vi "FGV.vi"(8 "error out 2":errorcluster, 10 "Write Data":T1, 11 "Enum":T5) -> (0 "error out":errorcluster, 3 "Read Data":T1)   [LabVIEW 2015, in "Copy of Untitled Library 1.lvlib"]
uses:
  Copy of Untitled Library 1.lvlib
  Controls/Enum Constant.ctl
  Controls/FGV Data.ctl
  Controls/FGV Cluster Data.ctl
  <userlib>/origin_lib_main/userlogin_lib/Control/Queue and Caller MSG.ctl
  <vilib>/addons/database/Connection.llb/Conn ObjectReference.ctl
  <vilib>/addons/database/NI_Database_API.lvlib
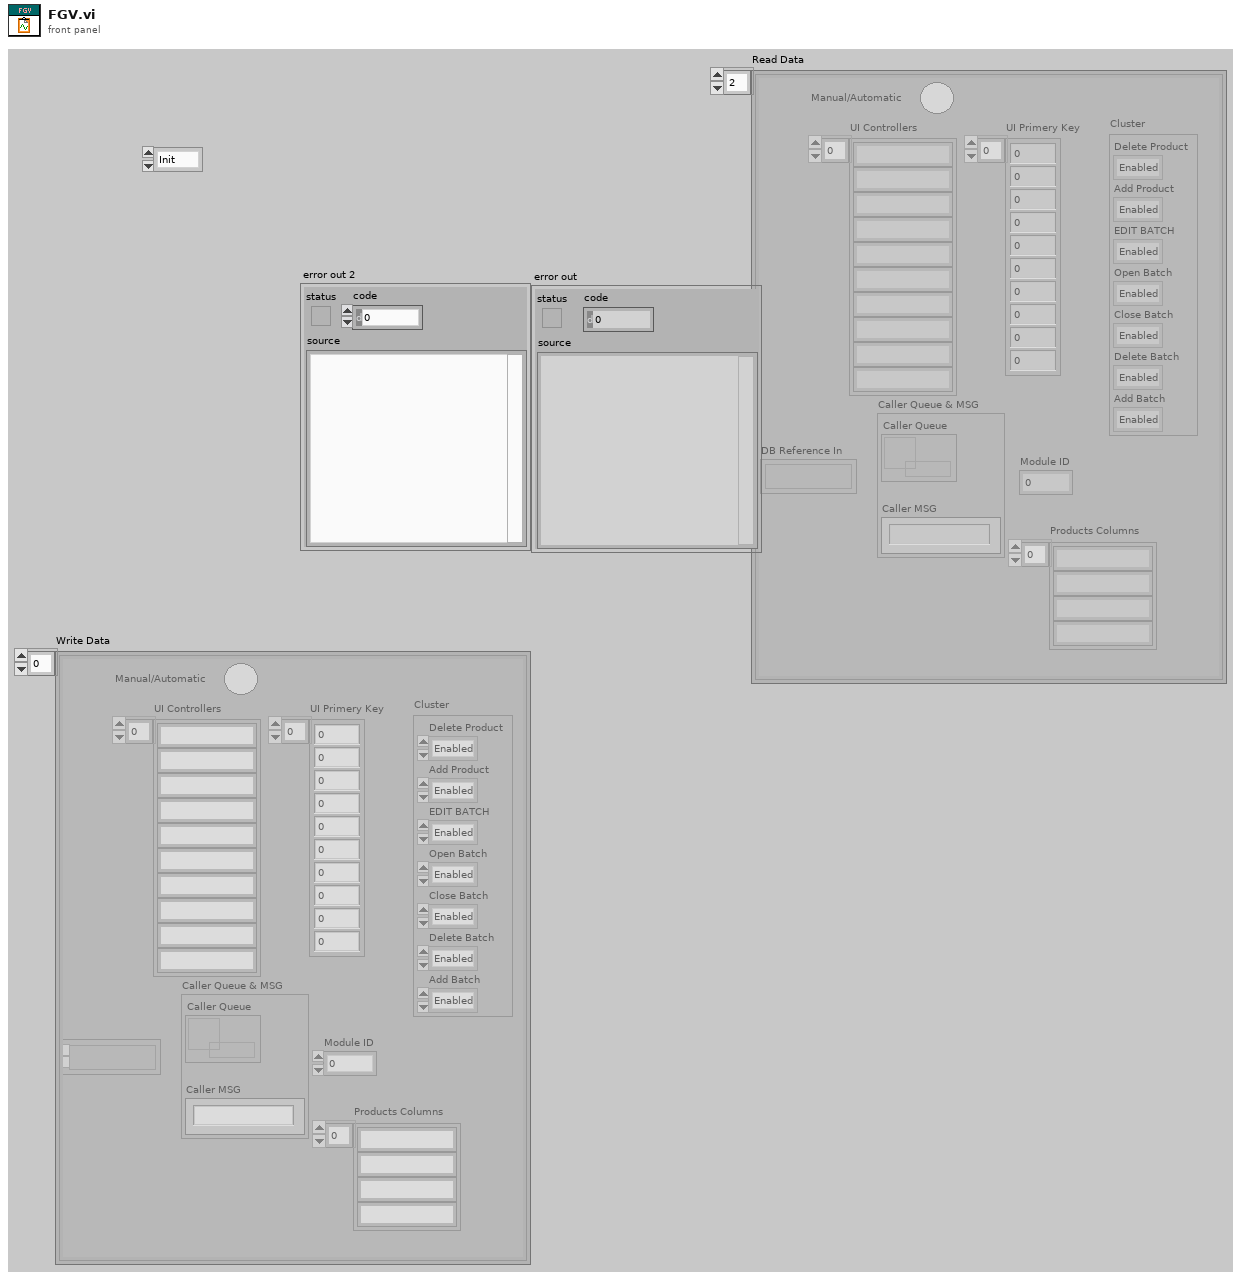
[diagram p1: front panel]
types:
  T1 = typedef "FGV Data.ctl" = T2[]
  T2 = typedef "FGV Cluster Data.ctl" = cluster{"Manual/Automatic":bool, "UI Controllers ":string[], "UI Primery Key ":dbl[], "Caller Queue & MSG":T3, "Module ID":dbl, "DB Reference In":T4, "Products Columns":string[], "Cluster":cluster{"Delete Product":enum8{"Enabled", "Disabled", "Disabled and Grayed Out"}, "Add Product ":enum8{"Enabled", "Disabled", "Disabled and Grayed Out"}, "EDIT BATCH":enum8{"Enabled", "Disabled", "Disabled and Grayed Out"}, "Open Batch ":enum8{"Enabled", "Disabled", "Disabled and Grayed Out"}, "Close Batch":enum8{"Enabled", "Disabled", "Disabled and Grayed Out"}, "Delete Batch":enum8{"Enabled", "Disabled", "Disabled and Grayed Out"}, "Add Batch ":enum8{"Enabled", "Disabled", "Disabled and Grayed Out"}}}
  T3 = typedef "Queue and Caller MSG.ctl" = cluster{"Caller Queue":refnum<queue>, "Caller MSG":string}
  T4 = typedef "NI_Database_API.lvlib/Conn ObjectReference.ctl" = refnum<k1>
  T5 = typedef "Enum Constant.ctl" = enum16{"Init", "Read", "Write"}
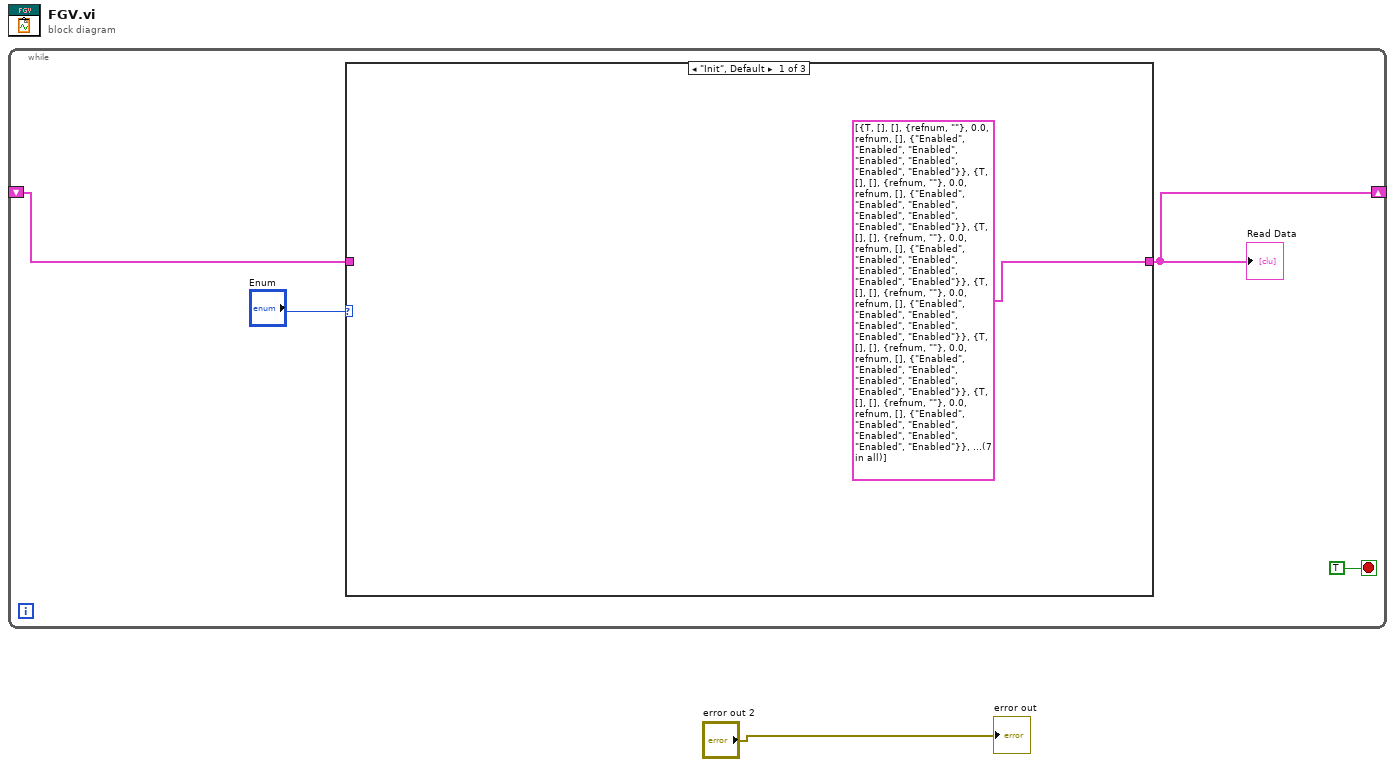
[diagram p0: block diagram]
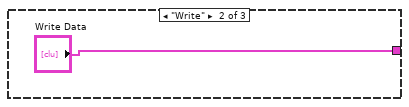
[diagram p2: hidden frame]
diagram:
  n1 = while {
    shift-right: [w3] -> _
    shift-left: _ -> [w2]
    stop <- TRUE stop-if-true
    n2 = case shown="\"Init\", Default" "Enum" {
      tunnel: [T1 [{"Manual/Automatic"=TRUE, "UI Controllers "=[], "UI Primery Key "=[], "Caller Queue & MSG"={"Caller Queue"=refnum, "Caller MSG"=""}, "Module ID"=0.0, "DB Reference In"=refnum, "Products Columns"=[], "Cluster"={"Delete Product"=enum."Enabled", "Add Product "=enum."Enabled", "EDIT BATCH"=enum."Enabled", "Open Batch "=enum."Enabled", "Close Batch"=enum."Enabled", "Delete Batch"=enum."Enabled", "Add Batch "=enum."Enabled"}}, {"Manual/Automatic"=TRUE, "UI Controllers "=[], "UI Primery Key "=[], "Caller Queue & MSG"={"Caller Queue"=refnum, "Caller MSG"=""}, "Module ID"=0.0, "DB Reference In"=refnum, "Products Columns"=[], "Cluster"={"Delete Product"=enum."Enabled", "Add Product "=enum."Enabled", "EDIT BATCH"=enum."Enabled", "Open Batch "=enum."Enabled", "Close Batch"=enum."Enabled", "Delete Batch"=enum."Enabled", "Add Batch "=enum."Enabled"}}, {"Manual/Automatic"=TRUE, "UI Controllers "=[], "UI Primery Key "=[], "Caller Queue & MSG"={"Caller Queue"=refnum, "Caller MSG"=""}, "Module ID"=0.0, "DB Reference In"=refnum, "Products Columns"=[], "Cluster"={"Delete Product"=enum."Enabled", "Add Product "=enum."Enabled", "EDIT BATCH"=enum."Enabled", "Open Batch "=enum."Enabled", "Close Batch"=enum."Enabled", "Delete Batch"=enum."Enabled", "Add Batch "=enum."Enabled"}}, {"Manual/Automatic"=TRUE, "UI Controllers "=[], "UI Primery Key "=[], "Caller Queue & MSG"={"Caller Queue"=refnum, "Caller MSG"=""}, "Module ID"=0.0, "DB Reference In"=refnum, "Products Columns"=[], "Cluster"={"Delete Product"=enum."Enabled", "Add Product "=enum."Enabled", "EDIT BATCH"=enum."Enabled", "Open Batch "=enum."Enabled", "Close Batch"=enum."Enabled", "Delete Batch"=enum."Enabled", "Add Batch "=enum."Enabled"}}, {"Manual/Automatic"=TRUE, "UI Controllers "=[], "UI Primery Key "=[], "Caller Queue & MSG"={"Caller Queue"=refnum, "Caller MSG"=""}, "Module ID"=0.0, "DB Reference In"=refnum, "Products Columns"=[], "Cluster"={"Delete Product"=enum."Enabled", "Add Product "=enum."Enabled", "EDIT BATCH"=enum."Enabled", "Open Batch "=enum."Enabled", "Close Batch"=enum."Enabled", "Delete Batch"=enum."Enabled", "Add Batch "=enum."Enabled"}}, {"Manual/Automatic"=TRUE, "UI Controllers "=[], "UI Primery Key "=[], "Caller Queue & MSG"={"Caller Queue"=refnum, "Caller MSG"=""}, "Module ID"=0.0, "DB Reference In"=refnum, "Products Columns"=[], "Cluster"={"Delete Product"=enum."Enabled", "Add Product "=enum."Enabled", "EDIT BATCH"=enum."Enabled", "Open Batch "=enum."Enabled", "Close Batch"=enum."Enabled", "Delete Batch"=enum."Enabled", "Add Batch "=enum."Enabled"}}, {"Manual/Automatic"=TRUE, "UI Controllers "=[], "UI Primery Key "=[], "Caller Queue & MSG"={"Caller Queue"=refnum, "Caller MSG"=""}, "Module ID"=0.0, "DB Reference In"=refnum, "Products Columns"=[], "Cluster"={"Delete Product"=enum."Enabled", "Add Product "=enum."Enabled", "EDIT BATCH"=enum."Enabled", "Open Batch "=enum."Enabled", "Close Batch"=enum."Enabled", "Delete Batch"=enum."Enabled", "Add Batch "=enum."Enabled"}}] ("Write Data") "Write Data" w8] -> w3
      tunnel: w2 -> [_ _ w8]
      frame "Init", Default {
      }
      frame "Write" {
      }
      frame "Read" {
      }
    }
    "Read Data" <- w3
  }
  "error out" <- "error out 2"
